vi "MBconvertDecimal.vi"(9 "Values":dbl[](array[numeric]) max=247.0 format="%.2f", 10 "Decimal points":u8[](array[numeric]) max=4, 11 "From (F) / to (T) decimal":bool) -> (1 "New values":dbl[](array[numeric]) max=247.0 format="%.2f")   [LabVIEW 2010]
doc: "VI converts from or to decimal, with respect to the number of decimal digits.\n\n\nExample: \n\nRead (convert from decimal)\nIf your modbus instrument replies with 271 and the instrument is setup with decimal digit 1, you should do the same in your software, because modbus only handles 16-bit words.\nUse this VI to convert it to 27.1\n\nWrite (convert to decimal)\nIf you want to use digits to set a register, convert it so that modbus interpretes it as a 16-bit word. 27.1 is 271 in Modbus.\n\nNote:\nIf Decimal points array is empty, all decimal points equals to zero. \nIf Length of Decimal point - array is smaller than length of Values - array, all remaining Decimal points in array equals to last value in Decimal point - array."
panel:
  # "From"
  # "To"
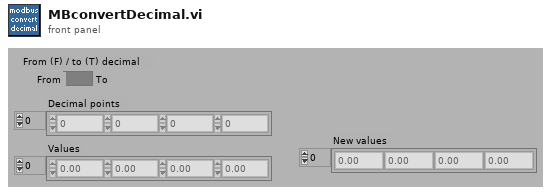
[diagram p1: front panel]
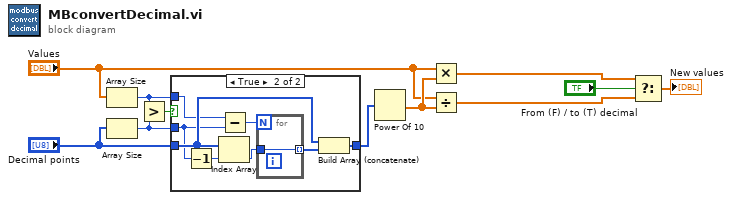
[diagram p0: block diagram]
diagram:
  n1 = Array Size(array="Values") -> (size(s)=w2:i32)
  n2 = Array Size(array="Decimal points") -> (size(s)=w1:i32)
  n3 = Greater?(x=w2, y=w1) -> (0:w6:bool)
  n4 = case shown="True" w6 {
    tunnel: "Decimal points" -> [w12 w18]
    tunnel: [w12 w19] -> w4
    tunnel: w1 -> [_ w14]
    tunnel: w2 -> [_ w15]
    frame False {
    }
    frame True {
      n5 = Decrement(x=w14) -> (x-1=w20:i32)
      n6 = Index Array(array=w18, index=w20) -> (element=w17:u8)
      n7 = Subtract(x=w15, y=w14) -> (x-y=w13:i32)
      n8 = for {
        N: w13 -> [_]
        tunnel: [w21] -> w16 mode=indexing
        tunnel: w17 -> [w21]
      }
      n9 = Build Array (concatenate)(w18, w16) -> (w19:u8[])
    }
  }
  n10 = Power Of 10(x=w4) -> (10^x=w7:dbl[])
  n11 = Multiply(x="Values", y=w7) -> (x*y=w10:dbl[])
  n12 = Divide(x="Values", y=w7) -> (x/y=w9:dbl[])
  n13 = Select(t=w10, s="From (F) / to (T) decimal", f=w9) -> (s? t:f=→"New values":dbl[])
